vi "Get - NT Enum.vi"(7 "PV name":string, 8 "error in (no error)":errorcluster, 9 "timeout":dbl[unit]=1.0, 10 "default":refnum<class "NT Enum.lvclass">, 11 "Client in":refnum<class "Client.lvclass">) -> (0 "error out":errorcluster, 1 "timed out?":bool, 2 "value":refnum<class "NT Enum.lvclass">, 3 "Client out":refnum<class "Client.lvclass">)   [LabVIEW 2020, in "PV Access.lvlib" / "PVA Client.lvlib" / "Client.lvclass"]
uses:
  Client.lvclass
  PV Data/NT Enum/NT Enum.lvclass
  C:/Users/eyw68381/source/repos/pvaccess-labview/labview/source/PV Data/Base/Base.lvclass
  PV Data/PV Data/PV Data.lvclass
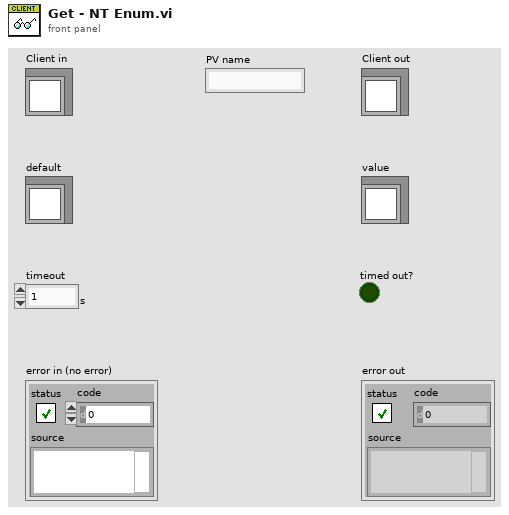
[diagram p1: front panel]
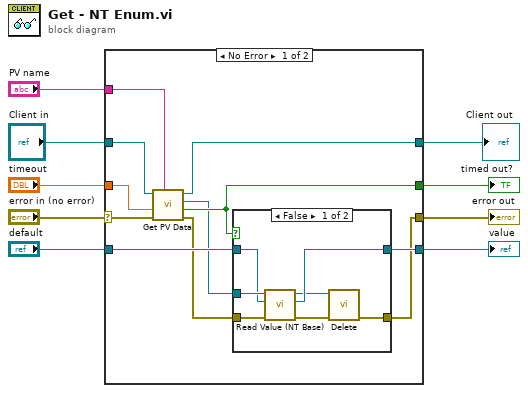
[diagram p0: block diagram]
diagram:
  n1 = case shown="No Error" "error in (no error)" {
    selector: "error in (no error)" -> [w13 w32]
    tunnel: [w12 w32] -> w2
    tunnel: [w14 w31] -> w4
    tunnel: "Client in" -> [w15 w31]
    tunnel: "default" -> [w20 w30]
    tunnel: [w19 w30] -> w1
    tunnel: "timeout" -> [w18 _]
    tunnel: [w17 _] -> w3
    tunnel: "PV name" -> [w16 _]
    frame No Error {
      n2 = call "Get PV Data.vi"("PV name"=w16, "error in"=w13, "timeout"=w18, "Client in"=w15) -> ("error out"=w10:errorcluster, "timed out?"=w17:bool, "PV Data out"=w11:refnum<class "PV Data.lvclass">, "Client out"=w14:refnum<class "Client.lvclass">)  [unwired: 4 in]
      n3 = case shown="False" w17 {
        tunnel: w10 -> [w26 w29]
        tunnel: w11 -> [w25 _]
        tunnel: [w27 w29] -> w12
        tunnel: [w23 w28] -> w19
        tunnel: w20 -> [w24 w28]
        frame False {
          n4 = call "Read Value (NT Base).vi"("error in (no error)"=w26, "default value"=w24, "PV Data in"=w25) -> ("error out"=w22:errorcluster, "value"=w23:refnum<class "NT Enum.lvclass">, "PV Data out"=w21:refnum<class "PV Data.lvclass">)  [unwired: 6 in]
          n5 = call "Delete.vi"("error in (no error)"=w22, "PV Data in"=w21) -> ("error out"=w27:errorcluster)  [unwired: 9 in]
        }
        frame True {
        }
      }
    }
    frame Error {
    }
  }
  "error out" <- w2
  "Client out" <- w4
  "value" <- w1
  "timed out?" <- w3
